vi "niRFUtil MEAS Channel Statistics.vi"(0 "Center Frequency (Hz)":dbl[](array[numeric]) format="%^.3e", 5 "Bandwidth (Hz)":dbl[](array[numeric]) format="%^.3e") -> (4 "Center (Hz)":dbl format="%^.3e", 6 "Span (Hz)":dbl format="%^.3e", 8 "Left Edge (Hz)":dbl format="%^.3e", 10 "Right Edge (Hz)":dbl format="%^.3e")   [LabVIEW 2015, in "niRFUtil.lvlib"]
uses:
  niRFUtil.lvlib
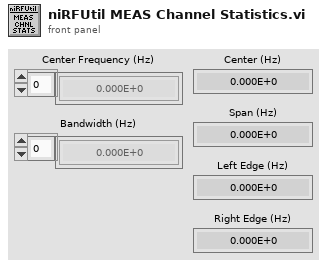
[diagram p1: front panel]
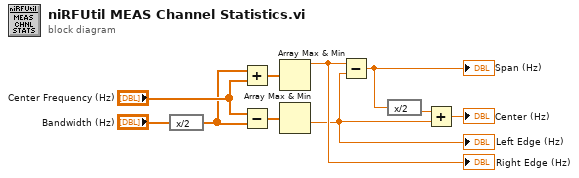
[diagram p0: block diagram]
diagram:
  n1 = expression code="x/2"("Bandwidth (Hz)") -> (w1:dbl[])
  n2 = Add(x=w1, y="Center Frequency (Hz)") -> (x+y=w9:dbl[])
  n3 = Subtract(x="Center Frequency (Hz)", y=w1) -> (x-y=w8:dbl[])
  n4 = Array Max & Min(array=w9) -> (max value=w6:dbl)  [unwired: 3 out]
  "Right Edge (Hz)" <- w6
  n5 = Array Max & Min(array=w8) -> (min value=w5:dbl)  [unwired: 3 out]
  "Left Edge (Hz)" <- w5
  n6 = Subtract(x=w6, y=w5) -> (x-y=w4:dbl)
  "Span (Hz)" <- w4
  n7 = expression code="x/2"(w4) -> (w3:dbl)
  n8 = Add(x=w3, y=w5) -> (x+y=→"Center (Hz)":dbl)
